vi "Destroy Self.vi"(7 "Sender":refnum<class "Sender.lvclass">) -> (2 "Msg":refnum<class "Msg.lvclass">)   [LabVIEW 2025, in "jettl.lvlib" / "Destroy Self Msg.lvlib"]
uses:
  Destroy Self Msg.lvlib
  Destroy Self Msg/Destroy Self Msg.lvclass
  C:/git/jettl/src/jettl/jettl/Destroy Self Msg/Go To Destroy Msg/Destroy Self Msg.lvclass
  C:/git/jettl/src/jettl/jettl/Msg/Msg.lvclass
  Msg/Msg.lvclass
  Sender/Sender/Sender.lvclass
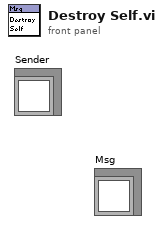
[diagram p1: front panel]
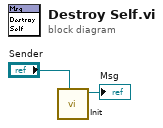
[diagram p0: block diagram]
diagram:
  n1 = call "Init.vi"("Sender"="Sender") -> ("Destroy Self Msg out"=→"Msg":refnum<class "Destroy Self Msg.lvclass">)  [unwired: 10 in]
